vi "LDO Bit Status Write.vi"(8 "error in":errorcluster, 11 "LDO Control Input":T1) -> (0 "error out":errorcluster, 3 "Bit Status":string[][](array[string]))   [LabVIEW 2020]
uses:
  Modbus/Modbus LDO Control.ctl
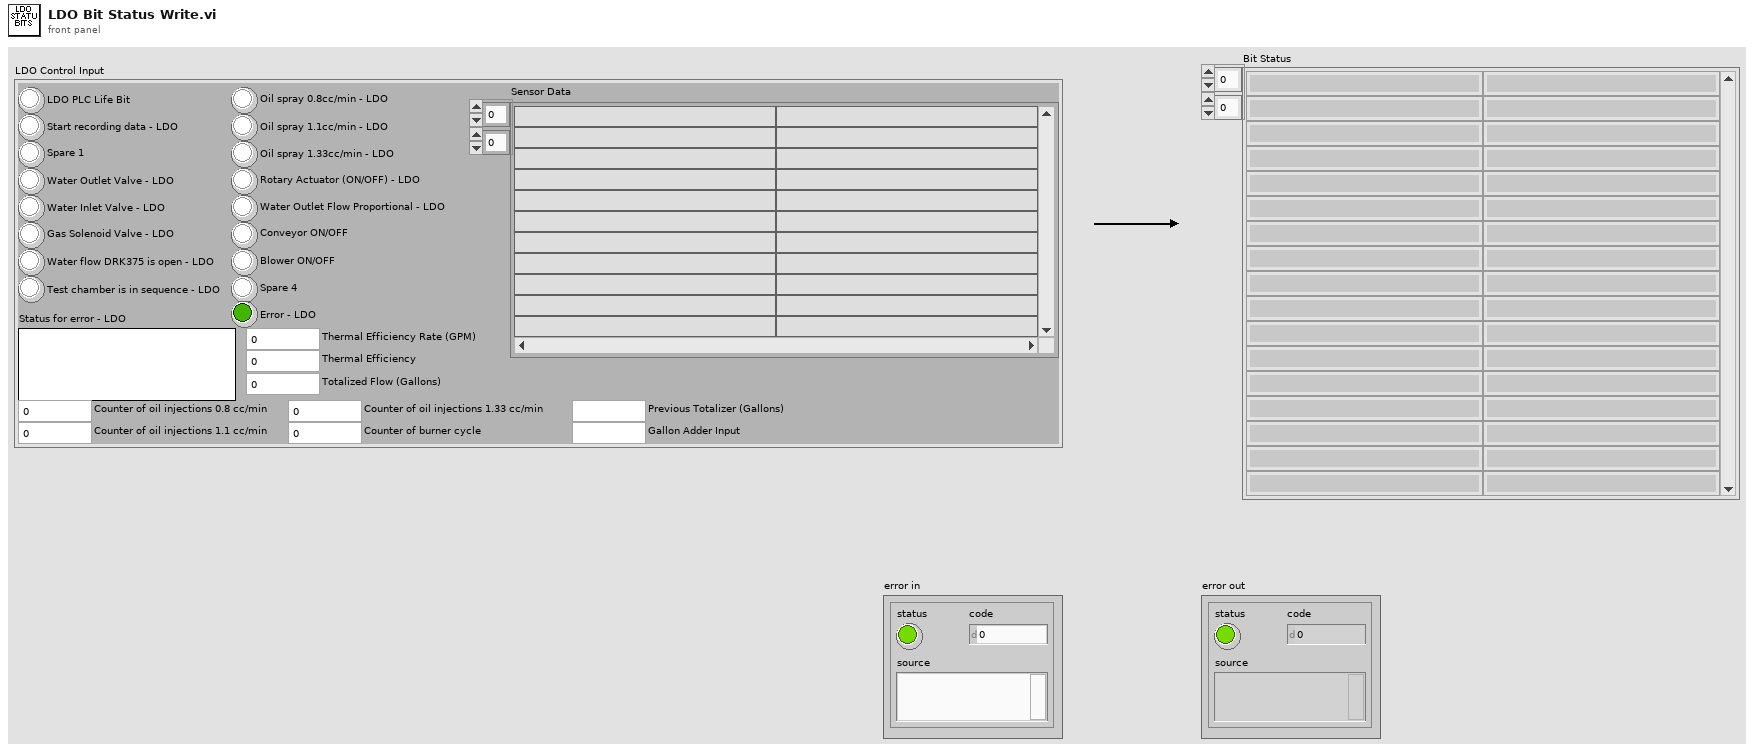
[diagram p1: front panel]
types:
  T1 = typedef "Modbus LDO Control.ctl" = cluster{"LDO PLC Life Bit":bool, "Start recording data - LDO":bool, "Spare 1":bool, "Water Outlet Valve - LDO":bool, "Water Inlet Valve - LDO":bool, "Gas Solenoid Valve - LDO":bool, "Water flow DRK375 is open - LDO":bool, "Test chamber is in sequence - LDO":bool, "Oil spray 0.8cc/min - LDO":bool, "Oil spray 1.1cc/min - LDO":bool, "Oil spray 1.33cc/min - LDO":bool, "Rotary Actuator (ON/OFF) - LDO":bool, "Water Outlet Flow Proportional - LDO":bool, "Conveyor ON/OFF":bool, "Blower ON/OFF":bool, "Spare 4":bool, "Status for error - LDO":string, "Error - LDO":bool, "Sensor Data":string[][], "Thermal Efficiency Rate (GPM)":dbl, "Thermal Efficiency":dbl, "Totalized Flow (Gallons)":dbl, "Counter of oil injections 1.33 cc/min":u16, "Counter of burner cycle":u16, "Counter of oil injections 1.1 cc/min":u16, "Counter of oil injections 0.8 cc/min":u16, "Previous Totalizer (Gallons)":dbl, "Gallon Adder Input":dbl}
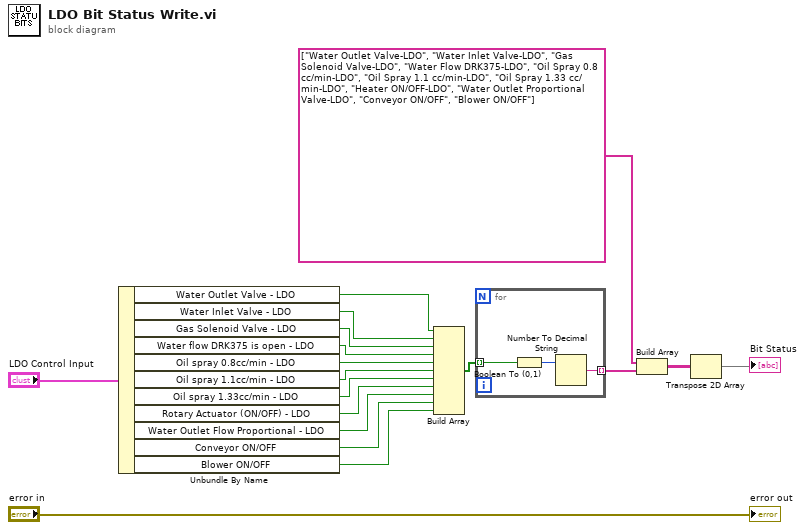
[diagram p0: block diagram]
diagram:
  n1 = Unbundle By Name("LDO Control Input") -> ("Water Outlet Valve - LDO"=w17:bool, "Water Inlet Valve - LDO"=w16:bool, "Gas Solenoid Valve - LDO"=w15:bool, "Water flow DRK375 is open - LDO"=w14:bool, "Oil spray 0.8cc/min - LDO"=w13:bool, "Oil spray 1.1cc/min - LDO"=w12:bool, "Oil spray 1.33cc/min - LDO"=w11:bool, "Rotary Actuator (ON/OFF) - LDO"=w10:bool, "Water Outlet Flow Proportional - LDO"=w9:bool, "Conveyor ON/OFF"=w2:bool, "Blower ON/OFF"=w1:bool)
  n2 = Build Array(w17, w16, w15, w14, w13, w12, w11, w10, w9, w2, w1) -> (w8:bool[])
  n3 = for {
    tunnel: w8 -> [w20] mode=indexing
    tunnel: [w19] -> w7 mode=indexing
    n4 = Boolean To (0,1)(Boolean=w20) -> (0, 1=w21:i16)
    n5 = Number To Decimal String(number=w21) -> (decimal integer string=w19:string)  [unwired: 1 in]
  }
  n6 = Build Array(string[] ["Water Outlet Valve-LDO", "Water Inlet Valve-LDO", "Gas Solenoid Valve-LDO", "Water Flow DRK375-LDO", "Oil Spray 0.8 cc/min-LDO", "Oil Spray 1.1 cc/min-LDO", "Oil Spray 1.33 cc/min-LDO", "Heater ON/OFF-LDO", "Water Outlet Proportional Valve-LDO", "Conveyor ON/OFF", "Blower ON/OFF"], w7) -> (w5:string[][])
  n7 = Transpose 2D Array(2D array=w5) -> (transposed array=→"Bit Status":string[][])
  "error out" <- "error in"
